vi "To JSON Tree.vi"(8 "error in (no error)":errorcluster, 11 "id in":refnum<class "id.lvclass">) -> (0 "error out":errorcluster, 2 "JSON out":refnum<class "JSON Null.lvclass">, 3 "id out":refnum<class "id.lvclass">)   [LabVIEW 2015, in "id.lvclass"]
uses:
  id.lvclass
  <vilib>/NI/JSON Support for LabVIEW/JSON Data Classes/JSON Datatype/JSON Null.lvclass
  id.lvclass/id.ctl
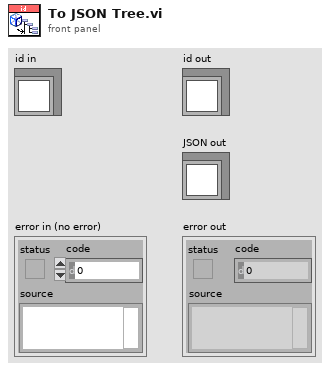
[diagram p1: front panel]
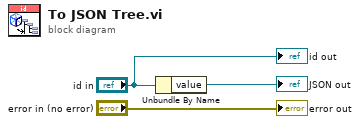
[diagram p0: block diagram]
diagram:
  n1 = Unbundle By Name("id in") -> ("value"=→"JSON out":refnum<class "JSON Null.lvclass">)
  "error out" <- "error in (no error)"
  "id out" <- "id in"
